vi "User Interface Component Test.vi"() -> ()   [LabVIEW 2017, in "DSF Core.lvlib"]
uses:
  DSF Core.lvlib
  Classes/User Interface/Core/Core User Interfaces.lvclass
  Classes/Component Configuration/Component Configurations.lvclass
  Components/Transceivers/UDP/Configuration/UDP Configurations.lvclass
  Components/Transceivers/UDP/UI/UDP Configuration User Interfaces.lvclass
  Classes/User Interface/Plugin/Component Settings Editor.lvclass
  C:/Git/DSF/Core/Classes/User Interface/User Interface.lvclass
  Classes/User Interface Handler/User Interface Handler.lvclass
  Classes/Component/Component.lvclass
  Classes/User Interface/User Interface.lvclass
panel:
  in  "stop":bool
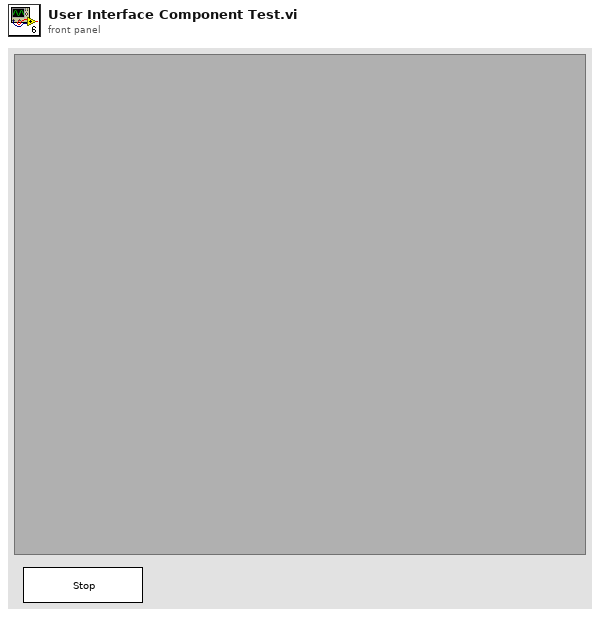
[diagram p1: front panel]
types:
  T1 = typedef "DSF Core.lvlib/User Interface Handler.lvclass/User Interface Ref.ctl" = refnum<vi>
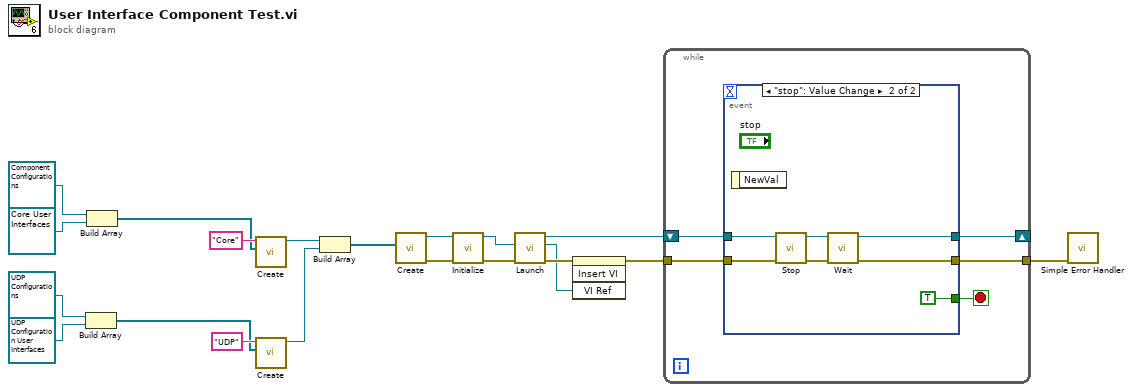
[diagram p0: block diagram]
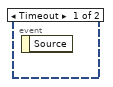
[diagram p2: hidden frame]
diagram:
  n1 = Build Array(refnum<class "UDP Configurations.lvclass"> refnum ("DSF Core.lvlib:UDP Configurations.lvclass"), refnum<class "UDP Configuration User Interfaces.lvclass"> refnum ("DSF Core.lvlib:UDP Configuration User Interfaces.lvclass")) -> (w10:refnum<class>[])
  n2 = Build Array(refnum<class "Component Configurations.lvclass"> refnum ("Configurations"), refnum<class "Core User Interfaces.lvclass"> refnum ("DSF Core.lvlib:Core Configuration UI.lvclass")) -> (w11:refnum<class>[])
  n3 = call "Create.vi"("objects"=w11, "name"="Core") -> ("Component"=w17:refnum<class "Component.lvclass">)  [unwired: 8 in, 1 out]
  n4 = call "Create.vi"("objects"=w10, "name"="UDP") -> ("Component"=w18:refnum<class "Component.lvclass">)  [unwired: 8 in, 1 out]
  n5 = Build Array(w17, w18) -> (w5:refnum<class "Component.lvclass">[])
  n6 = call "Create.vi"("Components"=w5) -> ("error out"=w6:errorcluster, "Component Settings Editor out"=w4:refnum<class "Component Settings Editor.lvclass">)  [unwired: 9 in]
  n7 = call-dynamic "Initialize.vi"("error in (no error)"=w6, "Component Settings Editor in"=w4) -> ("error out"=w3:errorcluster, "Component Settings Editor out"=w2:refnum<class "Component Settings Editor.lvclass">)  [unwired: 8 in]
  n8 = call "Launch.vi"("error in (no error)"=w3, "User Interface"=w2) -> ("error out"=w16:errorcluster, "active vi"=w14:T1, "User Interface Handler out"=w1:refnum<class "User Interface Handler.lvclass">)  [unwired: 7 in]
  n9 = invoke on="Sub Panel" class="SubPnl" method="Insert VI"(error in=w16, "VI Ref"=w14) -> (error out=w15:errorcluster)  [unwired: 2 in, 3 out]
  n10 = while {
    tunnel: w15 -> [w24]
    tunnel: [w23] -> w7
    shift-right: [w21] -> _
    shift-left: w1 -> [w22]
    stop <- w25 stop-if-true
    n11 = event shown="[1] \"stop\": Value Change" {
      selector: _ -> [_ _]
      dyn-events: _ -> [_ _]
      timeout: _ -> [_ _]
      tunnel: [_ TRUE] -> w25
      tunnel: w24 -> [_ w30]
      tunnel: [_ w27] -> w23
      tunnel: w22 -> [_ w29]
      tunnel: [_ w26] -> w21
      event Timeout {
        n12 = event-data() -> ()  [unwired: 1 in, 1 out]
      }
      event "stop": Value Change {
        n13 = event-data() -> ()  [unwired: 1 in, 1 out]
        n14 = call "Stop.vi"("error in (no error)"=w30, "User Interface Handler in"=w29) -> ("error out"=w31:errorcluster, "User Interface Handler out"=w28:refnum<class "User Interface Handler.lvclass">)  [unwired: 8 in]
        n15 = call "Wait.vi"("error in (no error)"=w31, "User Interface Handler in"=w28) -> ("error out"=w27:errorcluster, "User Interface Handler out"=w26:refnum<class "User Interface Handler.lvclass">)  [unwired: 7 in, 1 out]
      }
    }
  }
  n16 = call <vilib>:"Simple Error Handler.vi"("error in (no error)"=w7) -> ()  [unwired: 4 in, 5 out]
